vi "nm(j).vi"(4 "error in (no error)":errorcluster, 7 "j (1)":i32=1) -> (0 "error out":errorcluster, 1 "n":i32, 2 "m":i32, 3 "odd":bool)   [LabVIEW 2009, in "Zernike Polynome.lvlib"]
doc: "This VI searches the indices that correspond to the index j. Furthermore it returns whether j is even or odd."
uses:
  Zernike Polynome.lvlib
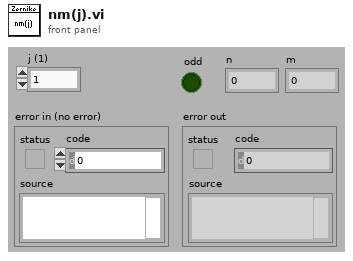
[diagram p1: front panel]
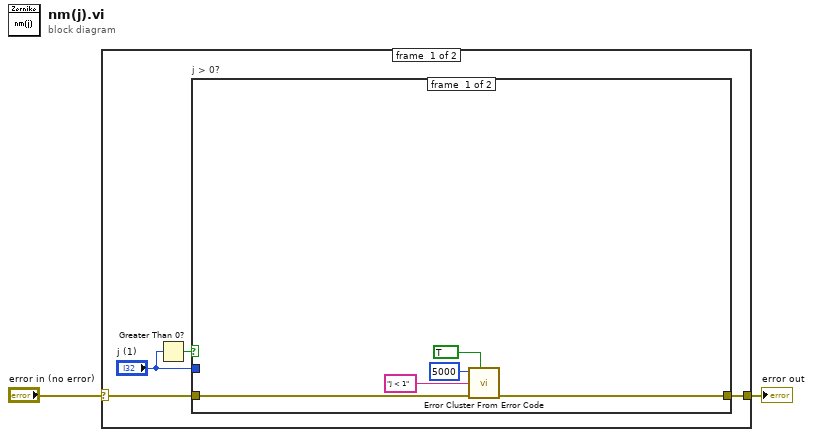
[diagram p0: block diagram]
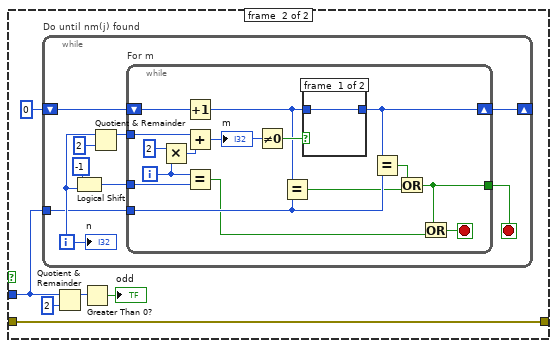
[diagram p2: hidden frame]
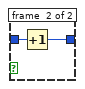
[diagram p3: hidden frame]
diagram:
  n1 = case shown="No Error" "error in (no error)" {
    selector: "error in (no error)" -> [w3 w46]
    tunnel: [w4 w46] -> w2
    frame #0 {
      n2 = Greater Than 0?(x="j (1)") -> (x > 0?=w5:bool)
      n3 = case "j > 0?" shown="True" w5 {
        tunnel: "j (1)" -> [_ w13]
        tunnel: w3 -> [w8 w12]
        tunnel: [w7 w12] -> w4
        frame #0 {
          n4 = call <vilib>:"Error Cluster From Error Code.vi"("show call chain? (False)"=TRUE, "error in (no error)"=w8, "error message (\"\")"="j < 1" ("error message (\"\")"), "error code (0)"=5000) -> ("error out"=w7:errorcluster)  [unwired: 5 in]
        }
        frame #1 {
          n5 = while "Do until nm(j) found" {
            shift-right: [w25] -> _
            shift-left: 0 -> [w26]
            tunnel: w13 -> [w19]
            i -> [w21]
            stop <- w18 stop-if-true
            n6 = Logical Shift(y=-1, x=w21) -> (x << y=w20:i32)
            n7 = Quotient & Remainder(x=w21, y=2) -> (x-y*floor(x/y)=w22:i32)  [unwired: 1 out]
            n8 = while "For m" {
              tunnel: w22 -> [w38]
              shift-right: [w34] -> w25
              shift-left: w26 -> [w40]
              tunnel: w20 -> [w35]
              tunnel: w19 -> [w31]
              tunnel: [w27] -> w18
              i -> [w36]
              stop <- w37 stop-if-true
              n9 = Multiply(x=2, y=w36) -> (x*y=w39:i32)
              n10 = Increment(x=w40) -> (x+1=w32:i32)
              n11 = Add(x=w38, y=w39) -> (x+y=w41:i32)
              "m" <- w41
              n12 = Equal?(x=w36, y=w35) -> (x = y?=w28:bool)
              n13 = Not Equal To 0?(x=w41) -> (x != 0?=w33:bool)
              n14 = Equal?(x=w32, y=w31) -> (x = y?=w29:bool)
              n15 = case shown="True" w33 {
                tunnel: w32 -> [w43 w45]
                tunnel: [w43 w44] -> w34
                frame #0 {
                }
                frame #1 {
                  n16 = Increment(x=w45) -> (x+1=w44:i32)
                }
              }
              n17 = Equal?(x=w34, y=w31) -> (x = y?=w30:bool)
              n18 = Or(x=w30, y=w29) -> (x .or. y?=w27:bool)
              n19 = Or(x=w27, y=w28) -> (x .or. y?=w37:bool)
            }
            "n" <- w21
          }
          n20 = Quotient & Remainder(x=w13, y=2) -> (x-y*floor(x/y)=w16:i32)  [unwired: 1 out]
          n21 = Greater Than 0?(x=w16) -> (x > 0?=→"odd":bool)
        }
      }
    }
    frame #1 {
    }
  }
  "error out" <- w2
